vi "氨氮质控流程.vi"(7 "队列输入NH3":refnum<queue>, 10 "氨氮":bool, 11 "氨氮量程切换":enum32{"H", "L", "AUTO"}(ring)=enum."AUTO") -> (2 "氨氮中断报警":bool, 3 "布尔":bool)   [LabVIEW 2016, in "质控单元.lvlib"]
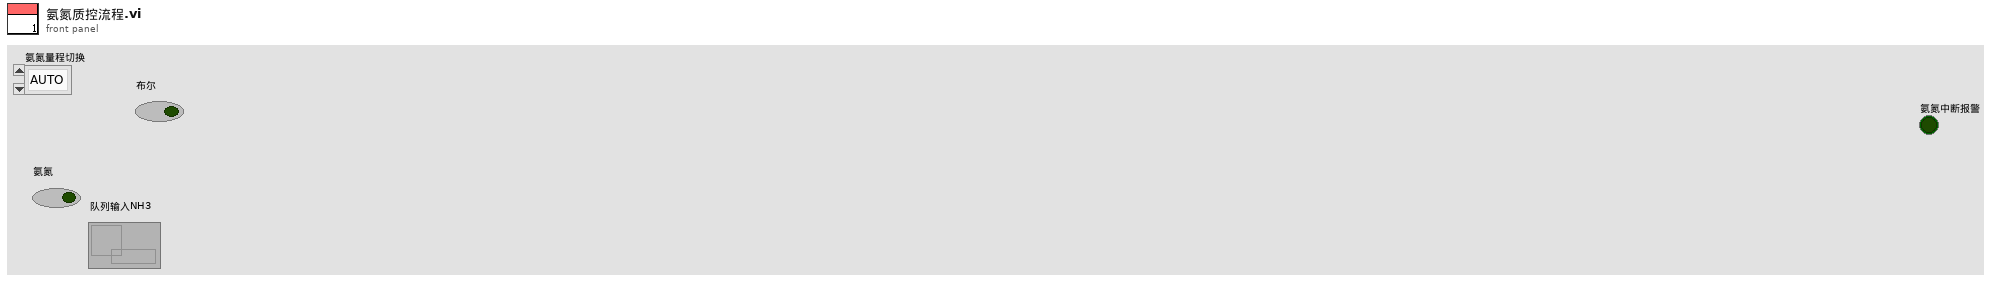
[diagram p1: front panel]
types:
  T1 = enum16{"待机", "启动氨氮水样", "氨氮测量中", "启动氨氮加标", "启动氨氮加标回收", "氨氮加标回收测量中", "启动总氮水样", "总氮测量中", "启动总氮加标", "启动总氮加标回收", "总氮加标回收测量中", "启动总磷水样", "总磷水样测量中", "启动总磷加标", "启动总磷加标回收", "总磷加标回收测量中", "结束"}
  T2 = cluster{"站号":u16, "量程切换":enum32{"H", "L", "AUTO"}, "控制命令":enum16{"启动测量", "标样核查", "零点核查", "跨度核查", "空白测试", "平行样测试", "加标回收", "空白校准", "标样校准", "初始化（清洗）", "停止测试", "仪器重启", "校时", "模式设置", "测量间隔设置"}, "模式设置":enum16{"待机", "连续模式", "周期模式", "定点模式", "受控模式", "手动模式"}, "测量间隔":u16}
  T3 = cluster{"时间标识":timestamp, "设备":string, "日志信息":string}
  T4 = cluster{"系统时间":timestamp, "工作状态":enum16{"空闲", "水样测试", "标样核查", "零点核查", "跨度核查", "空白测试", "平行样测试", "加标回收", "空白校准", "标样校准", "初始化（清洗）"}, "测量模式":enum16{"待机", "连续模式", "周期模式", "定点模式", "受控模式", "手动模式"}, "告警代码":enum16{"无告警", "缺试剂告警", "缺水样告警", "缺蒸馏水告警", "缺标液告警", "仪表漏液告警", "标定异常告警", "超量程告警", "加热异常", "低试剂预警", "超上限告警", "超下限告警", "仪表内部其他异常", "滴定异常告警", "电极异常告警", "量程切换告警", "参数设置告警", "PH电极电位异常", "电导率电极异常", "浊度光度异常", "溶解氧电极异常", "溶解氧光强异常", "温度异常告警", "PH异常告警", "溶解氧异常告警", "电导率异常告警", "浊度异常告警", "叶绿素异常告警", "藻密度异常告警", "蓝绿藻异常告警", "ORP异常告警", "氨氮异常告警", "清洁刷异常告警", "SD卡异常告警", "蓝牙异常告警", "Wifi异常告警", "流程异常告警"}, "故障代码":enum16{"无故障", "电机故障", "温度故障", "通讯故障", "滴定故障"}, "日志代码":u16, "软件版本":u16, "F0":sgl, "F1":sgl, "F2":sgl, "F3":sgl, "T":sgl, "H":sgl, "id":u16, "flowid":u16, "量程":u16}
  T5 = enum16{"空闲", "水样测试", "标样核查", "零点核查", "跨度核查", "空白测试", "平行样测试", "加标回收", "空白校准", "标样校准", "初始化（清洗）"}
  T6 = cluster{"因子编码":u32, "单位":u16, "标样参考值":sgl, "水样数据时间":timestamp, "水样实测值":sgl, "水样数据标识":string, "标样数据时间":timestamp, "标样实测值":sgl, "标样数据标识":string, "空白数据时间":timestamp, "空白实测值":sgl, "空白数据标识":string, "零点核查数据时间":timestamp, "零点核查实测值":sgl, "零点核查数据标识":string, "跨度核查数据时间":timestamp, "跨度核查实测值":sgl, "跨度核查数据标识":string, "加标回收数据时间":timestamp, "加标回收实测值":sgl, "加标回收数据标识":string, "平行样数据时间":timestamp, "平行样实测值":sgl, "平行样数据标识":string}
  T7 = cluster{"量程":dbl, "检出限":dbl, "加标前水样浓度":dbl, "加标后水样浓度":dbl, "加标水杯定容体积":dbl, "加标母液浓度":dbl, "加标体积":dbl, "加标回收率":dbl}
  T8 = cluster{"因子编码":u32, "单位":u16, "标样参考值":sgl, "水样数据时间":timestamp, "水样实测值":sgl, "水样数据标识":string, "标样数据时间":timestamp, "标样实测值":sgl, "标样数据标识":string, "空白数据时间":timestamp, "空白实测值":sgl, "空白数据标识":string, "零点核查数据时间":timestamp, "零点核查实测值":sgl, "零点核查数据标识":string, "跨度核查数据时间":timestamp, "跨度核查实测值":sgl, "跨度核查数据标识":string, "加标回收数据时间":timestamp, "加标回收实测值":sgl, "加标回收数据标识":string, "平行样数据时间":timestamp, "平行样实测值":sgl, "平行样数据标识":string, "F0":sgl, "F1":sgl, "F2":sgl, "F3":sgl, "F4":sgl, "F5":sgl, "F6":sgl, "F7":sgl, "温度":sgl, "湿度":sgl, "X值":sgl}
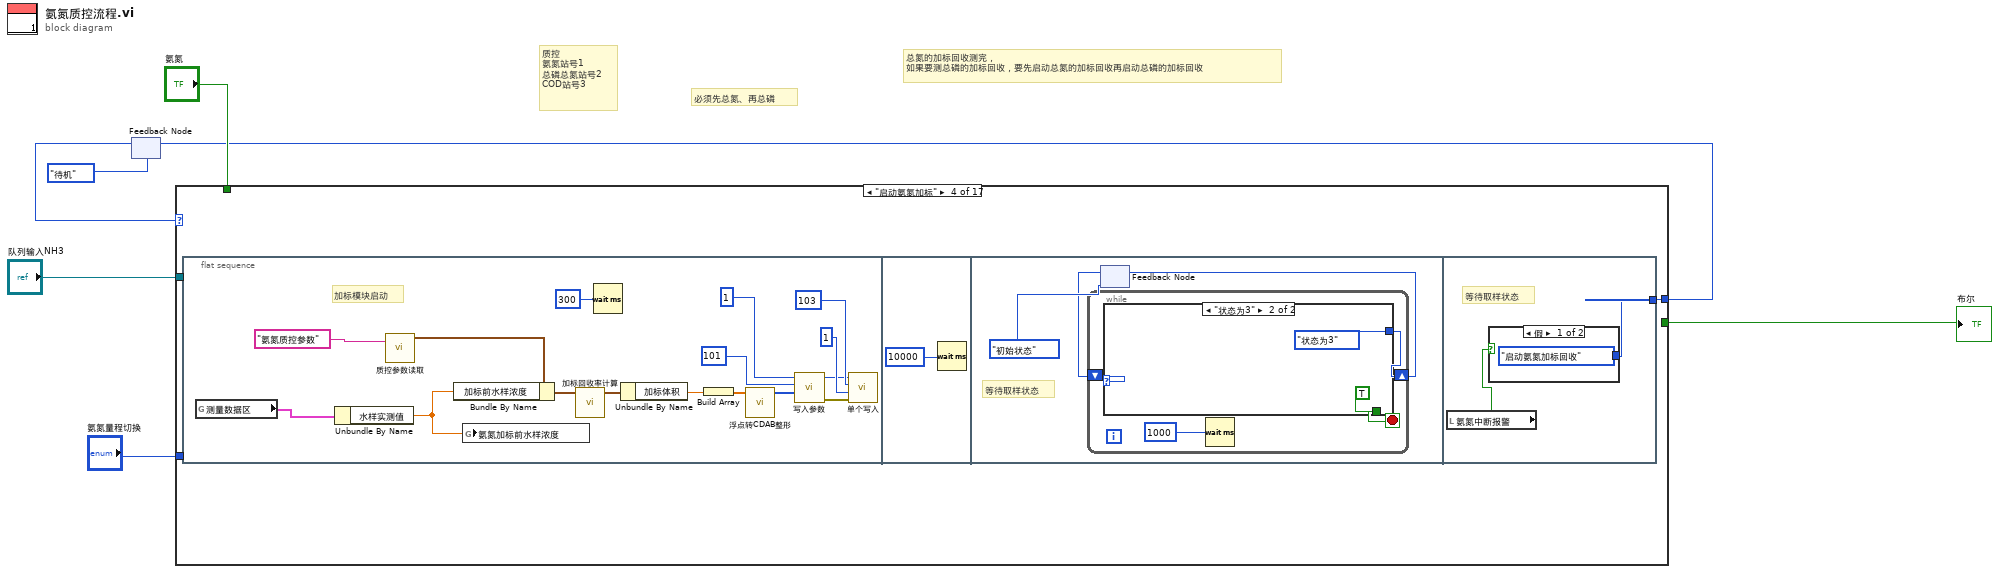
[diagram p0: block diagram]
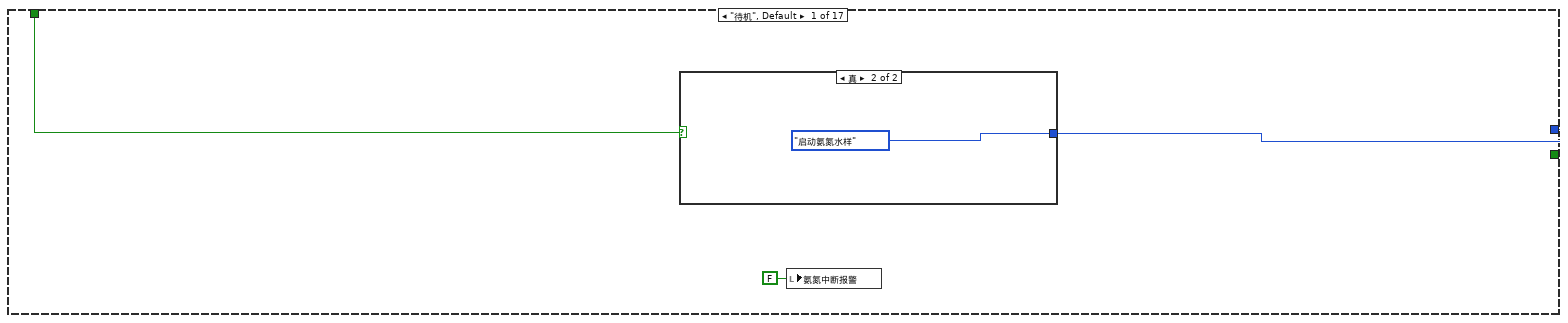
[diagram p2: hidden frame]
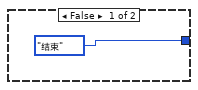
[diagram p3: hidden frame]
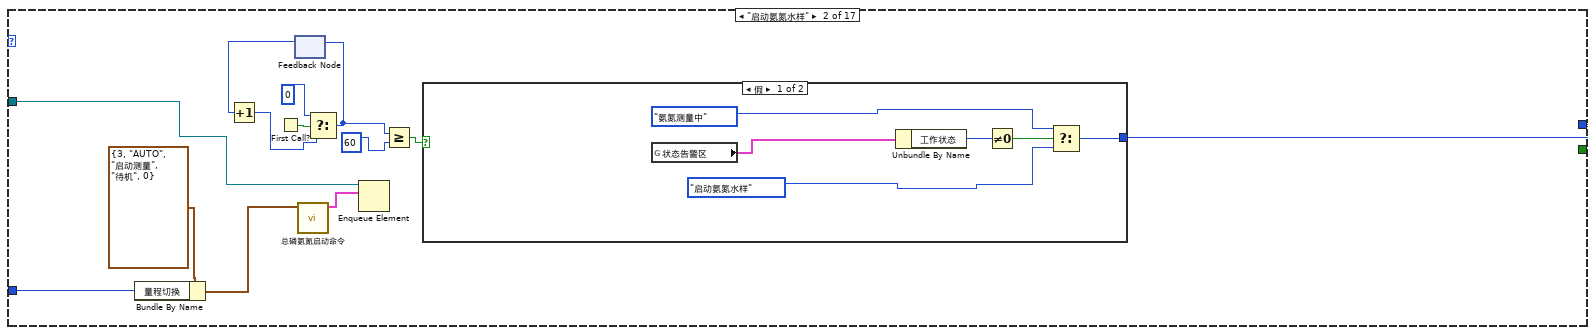
[diagram p4: hidden frame]
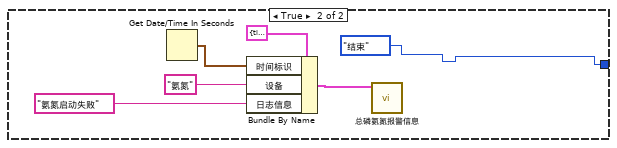
[diagram p5: hidden frame]
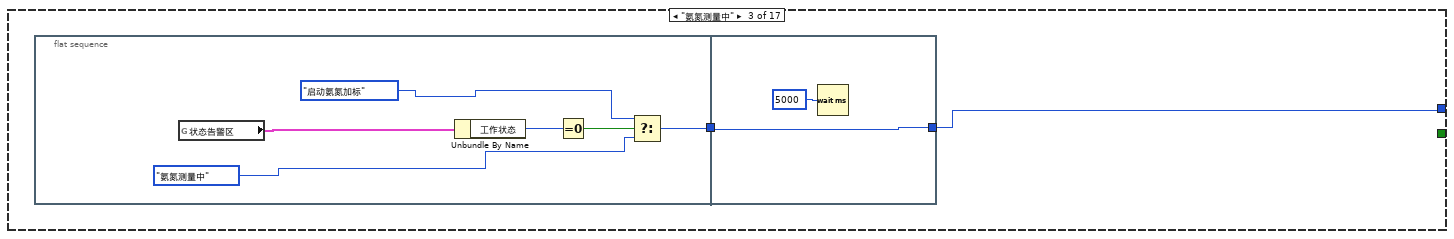
[diagram p6: hidden frame]
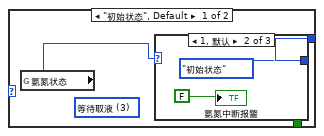
[diagram p7: hidden frame]
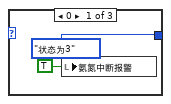
[diagram p8: hidden frame]
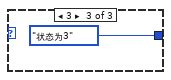
[diagram p9: hidden frame]
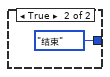
[diagram p10: hidden frame]
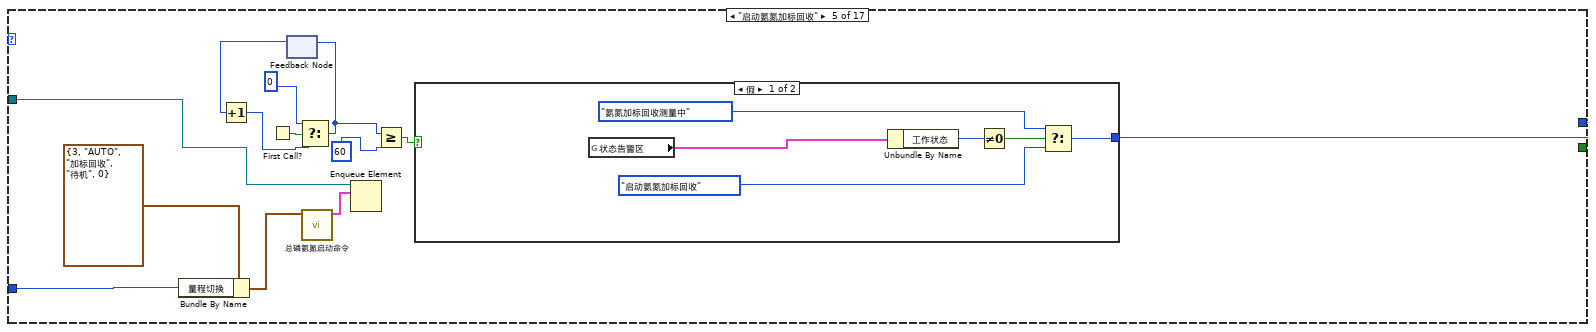
[diagram p11: hidden frame]
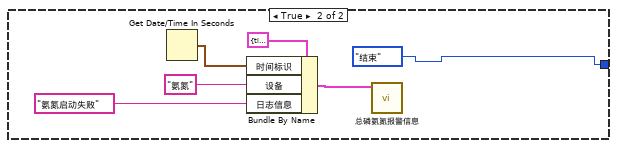
[diagram p12: hidden frame]
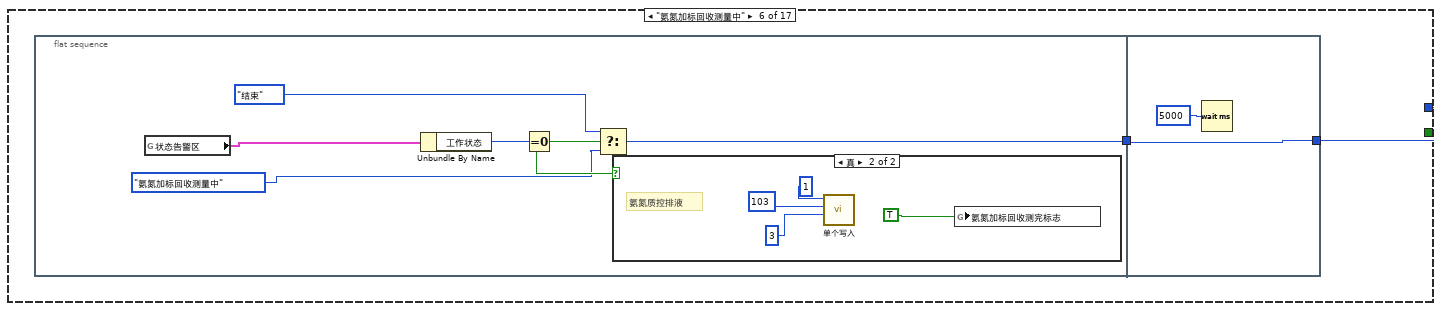
[diagram p13: hidden frame]
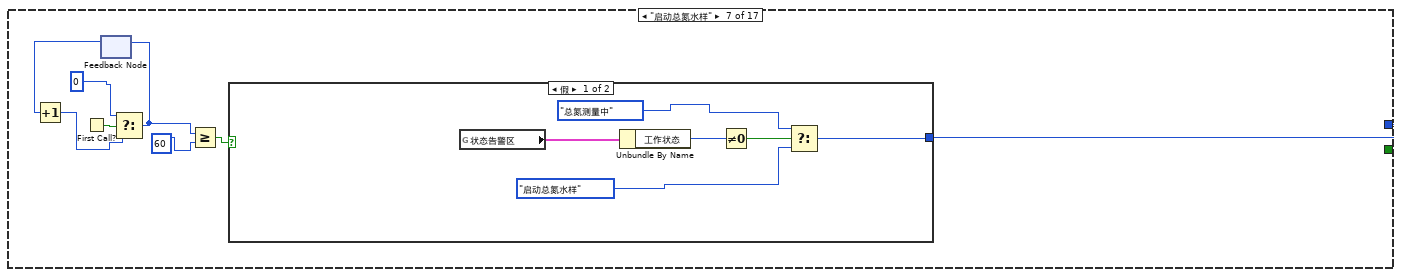
[diagram p15: hidden frame]
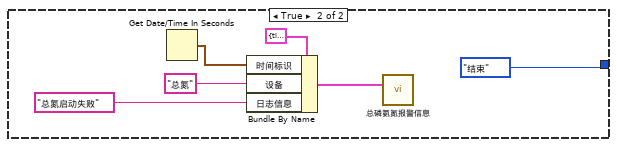
[diagram p16: hidden frame]
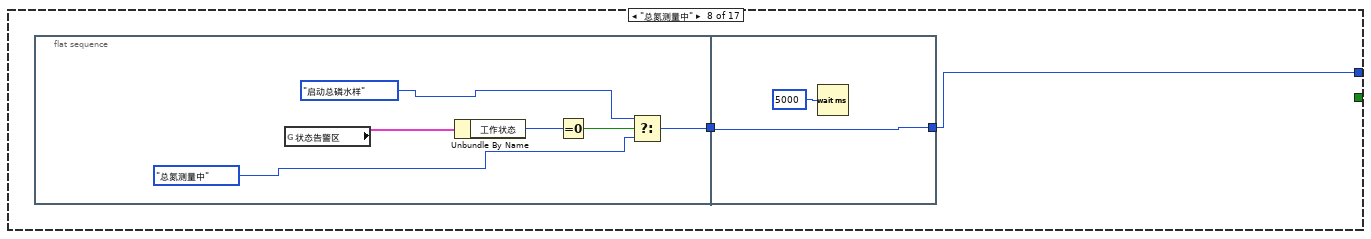
[diagram p17: hidden frame]
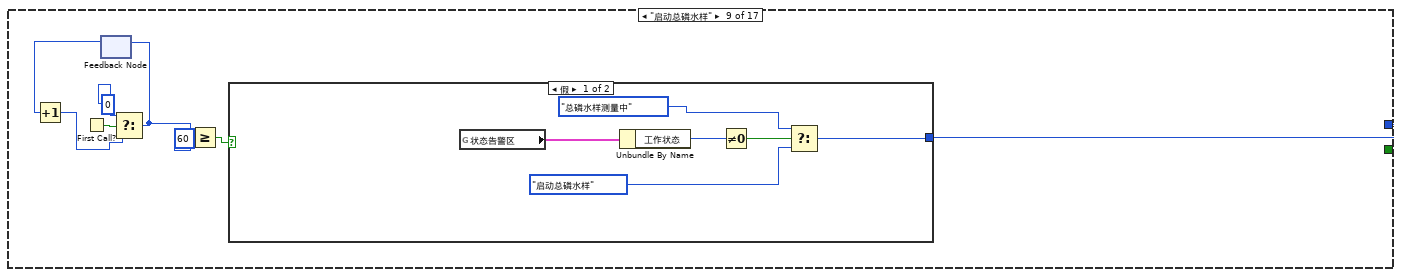
[diagram p18: hidden frame]
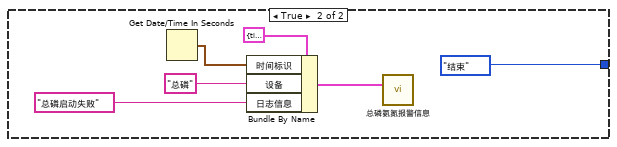
[diagram p19: hidden frame]
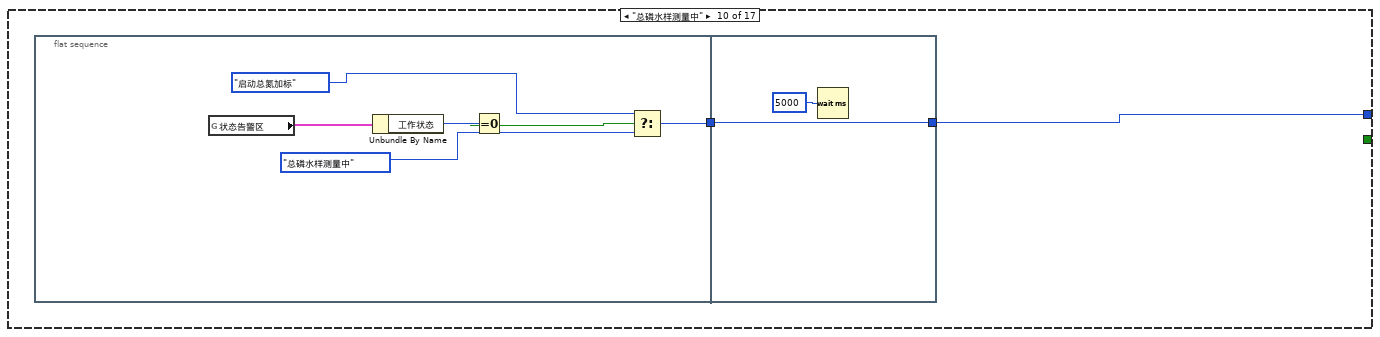
[diagram p20: hidden frame]
diagram:
  # "总氮的加标回收测完，\n如果要测总磷的加标回收，要先启动总氮的加标回收再启动总磷的加标回收"
  # "质控\n氨氮站号1   \n总磷总氮站号2\nCOD站号3"
  # "必须先总氮、再总磷"
  n1 = feedback #1(T1."待机") -> (w5:T1)
  n2 = case shown="\"启动氨氮加标\"" w5 {
    tunnel: [w10 w25 w39 w48 w90 w110 w131 w144 w161 w175 w184 w215 w235 w249 w280 w300 T1."结束"] -> w3
    tunnel: [_ _ _ _ _ _ _ _ _ _ _ _ _ _ _ _ TRUE] -> w6
    tunnel: "氨氮" -> [w9 _ _ _ _ _ _ _ _ _ _ _ _ _ _ _ _]
    tunnel: "队列输入NH3" -> [_ w16 _ _ w88 _ _ _ _ _ _ _ _ _ _ _ _]
    tunnel: "氨氮量程切换" -> [_ w13 _ _ w85 _ _ _ _ _ _ _ _ _ _ _ _]
    frame "待机", Default {
      n3 = case shown="真" w9 {
        tunnel: [T1."结束" T1."启动氨氮水样"] -> w10
        frame False {
        }
        frame True {
        }
      }
      n4 = local write "氨氮中断报警"(FALSE ("氨氮中断报警")) -> ()
    }
    frame "启动氨氮水样" {
      n5 = Bundle By Name(cluster=T2 {"站号"=3, "量程切换"=enum."AUTO", "控制命令"=enum."启动测量", "模式设置"=enum."待机", "测量间隔"=0} ("参数"), "量程切换"=w13) -> (w14:T2)
      n6 = First Call?() -> (First Call?: T/F=w23:bool)
      n7 = feedback #2() -> (w22:i32)  [unwired: 1 in]
      n8 = Increment(x=w22) -> (x+1=w21:i32)
      n9 = call "总磷氨氮启动命令.vi"("参数"=w14) -> ("启动命令"=w17:cluster{"命令":string, "data":variant})  [unwired: 10 in]
      n10 = Select(t=0, s=w23, f=w21) -> (s? t:f=w20:i32)
      n11 = feedback-in #2(w20) -> ()
      n12 = Enqueue Element(queue=w16, element=w17) -> ()  [unwired: 2 in, 3 out]
      n13 = Greater Or Equal?(x=w20, y=60) -> (x >= y?=w18:bool)
      n14 = case shown="假" w18 {
        tunnel: [w29 T1."结束"] -> w25
        frame False {
          n15 = global read "VAR总磷氨氮全局变量.vi" "状态告警区"() -> (w26:T4)
          n16 = Unbundle By Name(w26) -> ("工作状态"=w31:T5)
          n17 = Not Equal To 0?(x=w31) -> (x != 0?=w30:bool)
          n18 = Select(t=T1."氨氮测量中", s=w30, f=T1."启动氨氮水样") -> (s? t:f=w29:T1)
        }
        frame True {
          n19 = Get Date/Time In Seconds() -> (seconds since 1Jan1904=w37:timestamp)
          n20 = Bundle By Name(cluster=T3 {"时间标识"=timestamp(0 s since 1904-01-01), "设备"="", "日志信息"=""} ("data in"), "时间标识"=w37, "设备"="氨氮", "日志信息"="氨氮启动失败") -> (w33:T3)
          n21 = call "总磷氨氮报警信息.vi"("data in"=w33) -> ()  [unwired: 11 in]
        }
      }
    }
    frame "氨氮测量中" {
      n22 = flat-sequence {
        tunnel: [w44] -> w38
        tunnel: [w47] -> w39
        tunnel: w38 -> [w47]
        frame #0 {
          n23 = global read "VAR总磷氨氮全局变量.vi" "状态告警区"() -> (w40:T4)
          n24 = Unbundle By Name(w40) -> ("工作状态"=w45:T5)
          n25 = Equal To 0?(x=w45) -> (x = 0?=w43:bool)
          n26 = Select(t=T1."启动氨氮加标", s=w43, f=T1."氨氮测量中") -> (s? t:f=w44:T1)
        }
        frame #1 {
          n27 = Wait (ms)(milliseconds to wait=u32 5000 ("等待时间（毫秒）")) -> ()  [unwired: 1 out]
        }
      }
    }
    frame "启动氨氮加标" {
      n28 = flat-sequence {
        tunnel: [w82] -> w48
        frame #0 {
          w53 = u16 1 ("value")
          # "加标模块启动"
          n29 = global read "VAR总磷氨氮全局变量.vi" "测量数据区"() -> (w50:T6)
          n30 = Unbundle By Name(w50) -> ("水样实测值"=w51:sgl)
          n31 = call "质控参数读取.vi"("section"="氨氮质控参数") -> ("参数"=w61:T7)  [unwired: 9 in, 1 out]
          n32 = Bundle By Name(cluster=w61, "加标前水样浓度"=w51) -> (w62:T7)
          n33 = global write "水样浓度全局.vi" "氨氮加标前水样浓度"(w51) -> ()
          n34 = call "加标回收率计算.vi"("参数"=w62) -> ("参数 out"=w60:T7)  [unwired: 10 in]
          n35 = Wait (ms)(milliseconds to wait=u32 300 ("等待时间（毫秒）")) -> ()  [unwired: 1 out]
          n36 = Unbundle By Name(w60) -> ("加标体积"=w52:dbl)
          n37 = Build Array(w52) -> (w59:dbl[])
          n38 = call "浮点转CDAB整形.vi"("浮点数"=w59) -> ("CDAB整形输出"=w54:u16[])  [unwired: 10 in]
          n39 = call "写入参数.vi"("values"=w54, "starting address"=u16 101, "Slave ID"=w53) -> ("error out"=w58:errorcluster)  [unwired: 8 in]
          n40 = call "单个写入.vi"("Error in"=w58, "value"=u16 1, "address"=u16 103, "Slave ID"=w53) -> ()  [unwired: 7 in, 1 out]
        }
        frame #1 {
          n41 = Wait (ms)(milliseconds to wait=u32 10000 ("等待时间（毫秒）")) -> ()  [unwired: 1 out]
        }
        frame #2 {
          # "等待取样状态"
          n42 = feedback #3(enum16{"初始状态", "状态为3"}."初始状态") -> (w66:enum16{"初始状态", "状态为3"})
          n43 = while {
            shift-right: [w70] -> w65
            shift-left: w66 -> [w71]
            stop <- w69 stop-if-true
            n44 = case shown="\"状态为3\"" w71 {
              tunnel: [w73 enum16{"初始状态", "状态为3"}."状态为3"] -> w70
              tunnel: [_ TRUE] -> w69
              frame "初始状态", Default {
                (unwired) u16 3 items=["待机", "润洗", "进样", "等待取液", "排液"] ("氨氮状态")
                n45 = global read "氨氮加标回收状态全局变量.vi" "氨氮状态"() -> (w72:u16)
                n46 = case shown="1, 默认" w72 {
                  tunnel: [enum16{"初始状态", "状态为3"}."状态为3" enum16{"初始状态", "状态为3"}."初始状态" enum16{"初始状态", "状态为3"}."状态为3"] -> w73
                  frame 0 {
                    n47 = local write "氨氮中断报警"(TRUE ("氨氮中断报警")) -> ()
                  }
                  frame 1, Default {
                    "氨氮中断报警" <- FALSE ("总氮中断报警")
                  }
                  frame 3 {
                  }
                }
              }
              frame "状态为3" {
              }
            }
            n48 = Wait (ms)(milliseconds to wait=u32 1000 ("等待时间（毫秒）")) -> ()  [unwired: 1 out]
          }
          n49 = feedback-in #3(w65) -> ()
        }
        frame #3 {
          # "等待取样状态"
          n50 = local read "氨氮中断报警"() -> (w81:bool)
          n51 = case shown="假" w81 {
            tunnel: [T1."启动氨氮加标回收" T1."结束"] -> w82
            frame False {
            }
            frame True {
            }
          }
        }
      }
    }
    frame "启动氨氮加标回收" {
      n52 = Bundle By Name(cluster=T2 {"站号"=3, "量程切换"=enum."AUTO", "控制命令"=enum."加标回收", "模式设置"=enum."待机", "测量间隔"=0} ("参数"), "量程切换"=w85) -> (w86:T2)
      n53 = First Call?() -> (First Call?: T/F=w96:bool)
      n54 = feedback #4() -> (w95:i32)  [unwired: 1 in]
      n55 = Increment(x=w95) -> (x+1=w94:i32)
      n56 = Select(t=0, s=w96, f=w94) -> (s? t:f=w93:i32)
      n57 = feedback-in #4(w93) -> ()
      n58 = call "总磷氨氮启动命令.vi"("参数"=w86) -> ("启动命令"=w89:cluster{"命令":string, "data":variant})  [unwired: 10 in]
      n59 = Enqueue Element(queue=w88, element=w89) -> ()  [unwired: 2 in, 3 out]
      n60 = Greater Or Equal?(x=w93, y=60) -> (x >= y?=w91:bool)
      n61 = case shown="假" w91 {
        tunnel: [w101 T1."结束"] -> w90
        frame False {
          n62 = global read "VAR总磷氨氮全局变量.vi" "状态告警区"() -> (w98:T4)
          n63 = Unbundle By Name(w98) -> ("工作状态"=w103:T5)
          n64 = Not Equal To 0?(x=w103) -> (x != 0?=w102:bool)
          n65 = Select(t=T1."氨氮加标回收测量中", s=w102, f=T1."启动氨氮加标回收") -> (s? t:f=w101:T1)
        }
        frame True {
          n66 = Get Date/Time In Seconds() -> (seconds since 1Jan1904=w109:timestamp)
          n67 = Bundle By Name(cluster=T3 {"时间标识"=timestamp(0 s since 1904-01-01), "设备"="", "日志信息"=""} ("data in"), "时间标识"=w109, "设备"="氨氮", "日志信息"="氨氮启动失败") -> (w105:T3)
          n68 = call "总磷氨氮报警信息.vi"("data in"=w105) -> ()  [unwired: 11 in]
        }
      }
    }
    frame "氨氮加标回收测量中" {
      n69 = flat-sequence {
        tunnel: [w116] -> w111
        tunnel: [w123] -> w110
        tunnel: w111 -> [w123]
        frame #0 {
          n70 = global read "VAR总磷氨氮全局变量.vi" "状态告警区"() -> (w112:T4)
          n71 = Unbundle By Name(w112) -> ("工作状态"=w117:T5)
          n72 = Equal To 0?(x=w117) -> (x = 0?=w114:bool)
          n73 = Select(t=T1."结束", s=w114, f=T1."氨氮加标回收测量中") -> (s? t:f=w116:T1)
          n74 = case shown="真" w114 {
            frame False {
            }
            frame True {
              # "氨氮质控排液"
              n75 = call "单个写入.vi"("value"=u16 3, "address"=u16 103, "Slave ID"=u8 1) -> ()  [unwired: 8 in, 1 out]
              n76 = global write "质控测完标志全局 1.vi" "氨氮加标回收测完标志"(TRUE) -> ()
            }
          }
        }
        frame #1 {
          n77 = Wait (ms)(milliseconds to wait=u32 5000 ("等待时间（毫秒）")) -> ()  [unwired: 1 out]
        }
      }
    }
    frame "启动总氮水样" {
      n78 = First Call?() -> (First Call?: T/F=w129:bool)
      n79 = feedback #5() -> (w128:i32)  [unwired: 1 in]
      n80 = Increment(x=w128) -> (x+1=w127:i32)
      n81 = Select(t=0, s=w129, f=w127) -> (s? t:f=w126:i32)
      n82 = feedback-in #5(w126) -> ()
      n83 = Greater Or Equal?(x=w126, y=60) -> (x >= y?=w124:bool)
      n84 = case shown="假" w124 {
        tunnel: [w134 T1."结束"] -> w131
        frame False {
          n85 = global read "VAR总磷氨氮全局变量.vi" "状态告警区"() -> (w135:T4)
          n86 = Unbundle By Name(w135) -> ("工作状态"=w136:T5)
          n87 = Not Equal To 0?(x=w136) -> (x != 0?=w137:bool)
          n88 = Select(t=T1."总氮测量中", s=w137, f=T1."启动总氮水样") -> (s? t:f=w134:T1)
        }
        frame True {
          n89 = Get Date/Time In Seconds() -> (seconds since 1Jan1904=w143:timestamp)
          n90 = Bundle By Name(cluster=T3 {"时间标识"=timestamp(0 s since 1904-01-01), "设备"="", "日志信息"=""} ("data in"), "时间标识"=w143, "设备"="总氮", "日志信息"="总氮启动失败") -> (w139:T3)
          n91 = call "总磷氨氮报警信息.vi"("data in"=w139) -> ()  [unwired: 11 in]
        }
      }
    }
    frame "总氮测量中" {
      n92 = flat-sequence {
        tunnel: [w149] -> w145
        tunnel: [w153] -> w144
        tunnel: w145 -> [w153]
        frame #0 {
          n93 = global read "VAR总磷氨氮全局变量.vi" "状态告警区"() -> (w150:T4)
          n94 = Unbundle By Name(w150) -> ("工作状态"=w151:T5)
          n95 = Equal To 0?(x=w151) -> (x = 0?=w148:bool)
          n96 = Select(t=T1."启动总磷水样", s=w148, f=T1."总氮测量中") -> (s? t:f=w149:T1)
        }
        frame #1 {
          n97 = Wait (ms)(milliseconds to wait=u32 5000 ("等待时间（毫秒）")) -> ()  [unwired: 1 out]
        }
      }
    }
    frame "启动总磷水样" {
      n98 = First Call?() -> (First Call?: T/F=w159:bool)
      n99 = feedback #6() -> (w158:i32)  [unwired: 1 in]
      n100 = Increment(x=w158) -> (x+1=w157:i32)
      n101 = Select(t=0, s=w159, f=w157) -> (s? t:f=w156:i32)
      n102 = feedback-in #6(w156) -> ()
      n103 = Greater Or Equal?(x=w156, y=60) -> (x >= y?=w154:bool)
      n104 = case shown="假" w154 {
        tunnel: [w164 T1."结束"] -> w161
        frame False {
          n105 = global read "VAR总磷氨氮全局变量.vi" "状态告警区"() -> (w165:T4)
          n106 = Unbundle By Name(w165) -> ("工作状态"=w166:T5)
          n107 = Not Equal To 0?(x=w166) -> (x != 0?=w167:bool)
          n108 = Select(t=T1."总磷水样测量中", s=w167, f=T1."启动总磷水样") -> (s? t:f=w164:T1)
        }
        frame True {
          n109 = Get Date/Time In Seconds() -> (seconds since 1Jan1904=w173:timestamp)
          n110 = Bundle By Name(cluster=T3 {"时间标识"=timestamp(0 s since 1904-01-01), "设备"="", "日志信息"=""} ("data in"), "时间标识"=w173, "设备"="总磷", "日志信息"="总磷启动失败") -> (w169:T3)
          n111 = call "总磷氨氮报警信息.vi"("data in"=w169) -> ()  [unwired: 11 in]
        }
      }
    }
    frame "总磷水样测量中" {
      n112 = flat-sequence {
        tunnel: [w179] -> w174
        tunnel: [w183] -> w175
        tunnel: w174 -> [w183]
        frame #0 {
          n113 = global read "VAR总磷氨氮全局变量.vi" "状态告警区"() -> (w180:T4)
          n114 = Unbundle By Name(w180) -> ("工作状态"=w181:T5)
          n115 = Equal To 0?(x=w181) -> (x = 0?=w178:bool)
          n116 = Select(t=T1."启动总氮加标", s=w178, f=T1."总磷水样测量中") -> (s? t:f=w179:T1)
        }
        frame #1 {
          n117 = Wait (ms)(milliseconds to wait=u32 5000 ("等待时间（毫秒）")) -> ()  [unwired: 1 out]
        }
      }
    }
    frame "启动总氮加标" {
      n118 = flat-sequence {
        tunnel: [T1."启动总氮加标回收"] -> w184
        frame #0 {
          w189 = u16 2 ("value")
          # "加标模块启动"
          n119 = global read "VAR总磷氨氮全局变量.vi" "总氮测量数据区"() -> (w187:T8)
          n120 = Unbundle By Name(w187) -> ("水样实测值"=w185:sgl)
          n121 = call "质控参数读取.vi"("section"="总氮质控参数") -> ("参数"=w186:T7)  [unwired: 9 in, 1 out]
          n122 = Bundle By Name(cluster=w186, "加标前水样浓度"=w185) -> (w197:T7)
          n123 = global write "水样浓度全局.vi" "总氮加标前水样浓度"(w185) -> ()
          n124 = call "加标回收率计算.vi"("参数"=w197) -> ("参数 out"=w196:T7)  [unwired: 10 in]
          n125 = Unbundle By Name(w196) -> ("加标体积"=w188:dbl)
          n126 = Build Array(w188) -> (w195:dbl[])
          n127 = call "浮点转CDAB整形.vi"("浮点数"=w195) -> ("CDAB整形输出"=w190:u16[])  [unwired: 10 in]
          n128 = call "写入参数.vi"("values"=w190, "starting address"=u16 101, "Slave ID"=w189) -> ("error out"=w194:errorcluster)  [unwired: 8 in]
          n129 = call "单个写入.vi"("Error in"=w194, "value"=u16 2, "address"=u16 103, "Slave ID"=w189) -> ()  [unwired: 7 in, 1 out]
        }
        frame #1 {
          # "等待取样状态"
          n130 = feedback #7(enum16{"初始状态", "状态为3"}."初始状态") -> (w200:enum16{"初始状态", "状态为3"})
          n131 = while {
            shift-right: [w204] -> w199
            shift-left: w200 -> [w205]
            stop <- w203 stop-if-true
            n132 = case shown="\"初始状态\", 默认" w205 {
              tunnel: [w206 enum16{"初始状态", "状态为3"}."状态为3"] -> w204
              tunnel: [_ TRUE] -> w203
              frame "初始状态", Default {
                n133 = global read "氨氮加标回收状态全局变量.vi" "总磷状态"() -> (w208:u16)
                n134 = Equal?(x=w208, y=u16 3) -> (x = y?=w207:bool)
                n135 = case shown="真" w207 {
                  tunnel: [enum16{"初始状态", "状态为3"}."初始状态" enum16{"初始状态", "状态为3"}."状态为3"] -> w206
                  frame False {
                  }
                  frame True {
                  }
                }
              }
              frame "状态为3" {
              }
            }
            n136 = Wait (ms)(milliseconds to wait=u32 1000 ("等待时间（毫秒）")) -> ()  [unwired: 1 out]
          }
          n137 = feedback-in #7(w199) -> ()
        }
        frame #2 {
          # "等待取样状态"
        }
      }
    }
    frame "启动总氮加标回收" {
      n138 = First Call?() -> (First Call?: T/F=w221:bool)
      n139 = feedback #8() -> (w220:i32)  [unwired: 1 in]
      n140 = Increment(x=w220) -> (x+1=w219:i32)
      n141 = Select(t=0, s=w221, f=w219) -> (s? t:f=w218:i32)
      n142 = feedback-in #8(w218) -> ()
      n143 = Greater Or Equal?(x=w218, y=60) -> (x >= y?=w216:bool)
      n144 = case shown="假" w216 {
        tunnel: [w225 T1."结束"] -> w215
        frame False {
          n145 = global read "VAR总磷氨氮全局变量.vi" "状态告警区"() -> (w228:T4)
          n146 = Unbundle By Name(w228) -> ("工作状态"=w227:T5)
          n147 = Not Equal To 0?(x=w227) -> (x != 0?=w226:bool)
          n148 = Select(t=T1."启动总磷加标回收", s=w226, f=T1."启动总氮加标回收") -> (s? t:f=w225:T1)
        }
        frame True {
          n149 = Get Date/Time In Seconds() -> (seconds since 1Jan1904=w234:timestamp)
          n150 = Bundle By Name(cluster=T3 {"时间标识"=timestamp(0 s since 1904-01-01), "设备"="", "日志信息"=""} ("data in"), "时间标识"=w234, "设备"="总氮", "日志信息"="总氮启动失败") -> (w230:T3)
          n151 = call "总磷氨氮报警信息.vi"("data in"=w230) -> ()  [unwired: 11 in]
        }
      }
    }
    frame "总氮加标回收测量中" {
      n152 = flat-sequence {
        tunnel: [w240] -> w236
        tunnel: [w248] -> w235
        tunnel: w236 -> [w248]
        frame #0 {
          n153 = global read "VAR总磷氨氮全局变量.vi" "状态告警区"() -> (w241:T4)
          n154 = Unbundle By Name(w241) -> ("工作状态"=w242:T5)
          n155 = Equal To 0?(x=w242) -> (x = 0?=w238:bool)
          n156 = Select(t=T1."启动总磷加标", s=w238, f=T1."总氮加标回收测量中") -> (s? t:f=w240:T1)
          n157 = case shown="真" w238 {
            frame False {
            }
            frame True {
              # "总氮质控排液"
              n158 = call "单个写入.vi"("value"=u16 3, "address"=u16 103, "Slave ID"=u8 2) -> ()  [unwired: 8 in, 1 out]
              n159 = global write "质控测完标志全局 1.vi" "总氮加标回收测完标志"(TRUE) -> ()
            }
          }
        }
        frame #1 {
          n160 = Wait (ms)(milliseconds to wait=u32 5000 ("等待时间（毫秒）")) -> ()  [unwired: 1 out]
        }
      }
    }
    frame "启动总磷加标" {
      n161 = flat-sequence {
        tunnel: [T1."启动总氮加标回收"] -> w249
        frame #0 {
          w254 = u16 2 ("value")
          # "加标模块启动"
          n162 = global read "VAR总磷氨氮全局变量.vi" "测量数据区"() -> (w252:T8)
          n163 = Unbundle By Name(w252) -> ("水样实测值"=w250:sgl)
          n164 = call "质控参数读取.vi"("section"="总磷质控参数") -> ("参数"=w251:T7)  [unwired: 9 in, 1 out]
          n165 = Bundle By Name(cluster=w251, "加标前水样浓度"=w250) -> (w262:T7)
          n166 = global write "水样浓度全局.vi" "总磷加标前水样浓度"(w250) -> ()
          n167 = call "加标回收率计算.vi"("参数"=w262) -> ("参数 out"=w261:T7)  [unwired: 10 in]
          n168 = Unbundle By Name(w261) -> ("加标体积"=w253:dbl)
          n169 = Build Array(w253) -> (w260:dbl[])
          n170 = call "浮点转CDAB整形.vi"("浮点数"=w260) -> ("CDAB整形输出"=w255:u16[])  [unwired: 10 in]
          n171 = call "写入参数.vi"("values"=w255, "starting address"=u16 101, "Slave ID"=w254) -> ("error out"=w259:errorcluster)  [unwired: 8 in]
          n172 = call "单个写入.vi"("Error in"=w259, "value"=u16 2, "address"=u16 103, "Slave ID"=w254) -> ()  [unwired: 7 in, 1 out]
        }
        frame #1 {
          # "等待取样状态"
          n173 = feedback #9(enum16{"初始状态", "状态为3"}."初始状态") -> (w265:enum16{"初始状态", "状态为3"})
          n174 = while {
            shift-right: [w269] -> w264
            shift-left: w265 -> [w270]
            stop <- w268 stop-if-true
            n175 = case shown="\"状态为3\"" w270 {
              tunnel: [w271 enum16{"初始状态", "状态为3"}."状态为3"] -> w269
              tunnel: [_ TRUE] -> w268
              frame "初始状态", Default {
                n176 = global read "氨氮加标回收状态全局变量.vi" "总磷状态"() -> (w273:u16)
                n177 = Equal?(x=w273, y=u16 3) -> (x = y?=w272:bool)
                n178 = case shown="真" w272 {
                  tunnel: [enum16{"初始状态", "状态为3"}."初始状态" enum16{"初始状态", "状态为3"}."状态为3"] -> w271
                  frame False {
                  }
                  frame True {
                  }
                }
              }
              frame "状态为3" {
                (unwired) TRUE
              }
            }
            n179 = Wait (ms)(milliseconds to wait=u32 1000 ("等待时间（毫秒）")) -> ()  [unwired: 1 out]
          }
          n180 = feedback-in #9(w264) -> ()
        }
        frame #2 {
          # "等待取样状态"
        }
      }
    }
    frame "启动总磷加标回收" {
      n181 = First Call?() -> (First Call?: T/F=w286:bool)
      n182 = feedback #10() -> (w285:i32)  [unwired: 1 in]
      n183 = Increment(x=w285) -> (x+1=w284:i32)
      n184 = Select(t=0, s=w286, f=w284) -> (s? t:f=w283:i32)
      n185 = feedback-in #10(w283) -> ()
      n186 = Greater Or Equal?(x=w283, y=60) -> (x >= y?=w281:bool)
      n187 = case shown="假" w281 {
        tunnel: [w290 T1."结束"] -> w280
        frame False {
          n188 = global read "VAR总磷氨氮全局变量.vi" "状态告警区"() -> (w291:T4)
          n189 = Unbundle By Name(w291) -> ("工作状态"=w292:T5)
          n190 = Not Equal To 0?(x=w292) -> (x != 0?=w293:bool)
          n191 = Select(t=T1."总磷加标回收测量中", s=w293, f=T1."启动总磷加标回收") -> (s? t:f=w290:T1)
        }
        frame True {
          n192 = Get Date/Time In Seconds() -> (seconds since 1Jan1904=w299:timestamp)
          n193 = Bundle By Name(cluster=T3 {"时间标识"=timestamp(0 s since 1904-01-01), "设备"="", "日志信息"=""} ("data in"), "时间标识"=w299, "设备"="总磷", "日志信息"="总磷启动失败") -> (w295:T3)
          n194 = call "总磷氨氮报警信息.vi"("data in"=w295) -> ()  [unwired: 11 in]
        }
      }
    }
    frame "总磷加标回收测量中" {
      n195 = flat-sequence {
        tunnel: [w305] -> w301
        tunnel: [w313] -> w300
        tunnel: w301 -> [w313]
        frame #0 {
          n196 = global read "VAR总磷氨氮全局变量.vi" "状态告警区"() -> (w306:T4)
          n197 = Unbundle By Name(w306) -> ("工作状态"=w307:T5)
          n198 = Equal To 0?(x=w307) -> (x = 0?=w304:bool)
          n199 = Select(t=T1."结束", s=w304, f=T1."总磷加标回收测量中") -> (s? t:f=w305:T1)
          n200 = case shown="真" w304 {
            frame False {
            }
            frame True {
              # "总磷质控排液"
              n201 = global write "质控测完标志全局 1.vi" "总磷加标回收测完标志"(TRUE) -> ()
              n202 = call "单个写入.vi"("value"=u16 3, "address"=u16 103, "Slave ID"=u8 2) -> ()  [unwired: 8 in, 1 out]
            }
          }
        }
        frame #1 {
          n203 = Wait (ms)(milliseconds to wait=u32 5000 ("等待时间（毫秒）")) -> ()  [unwired: 1 out]
        }
      }
    }
    frame "结束" {
    }
  }
  "布尔" <- w6
  n204 = feedback-in #1(w3) -> ()
